vi "HEWH RLT PRAT.vi"() -> ()   [LabVIEW 2023] (continued)
"Condition#"=enum."C1", "Draw Flags"=enum."N/A", "Data Processing Delay (FHD 15sec, UEF 5 Sec)"=0.0, "Test Complete"=FALSE, "User Setpoint"=0.0, "Tank Setpoint"=0.0}, {"Sequence #"=6.0, "Cycles"=15, "Mode Setting"="", "Flow Rate (GPM)"=0.0, "Temperature (F)"=0.0, "Reset Timer"=FALSE, "Use Temp Decline Method"=FALSE, "Terminate Condition"=enum."C1-Terminate Draw @ Gallon Mark", "Condition Value #1"=0.0, "UE"=FALSE, "LE"=FALSE, "Comp"=FALSE, "Fan"=FALSE, "Test End Time (Sec)"=0.0, "Purge Until Cutout"=FALSE, "Start Conditions"=enum."Heat Source Cutout", "Condition Value #2"=0.0, "Remove Power"=FALSE, "Time"=0.0, "Check Special Cond."=enum."SC2-Check Heat Source (On-C2/Off-C1)", "Condition#"=enum."C1", "Draw Flags"=enum."N/A", "Data Processing Delay (FHD 15sec, UEF 5 Sec)"=0.0, "Test Complete"=FALSE, "User Setpoint"=0.0, "Tank Setpoint"=0.0}, {"Sequence #"=7.0, "Cycles"=35, "Mode Setting"="", "Flow Rate (GPM)"=0.0, "Temperature (F)"=0.0, "Reset Timer"=FALSE, "Use Temp Decline Method"=FALSE, "Terminate Condition"=enum."C1-Terminate Draw @ Gallon Mark", "Condition Value #1"=0.0, "UE"=FALSE, "LE"=FALSE, "Comp"=FALSE, "Fan"=FALSE, "Test End Time (Sec)"=0.0, "Purge Until Cutout"=FALSE, "Start Conditions"=enum."Heat Source Cutout", "Condition Value #2"=0.0, "Remove Power"=FALSE, "Time"=0.0, "Check Special Cond."=enum."SC2-Check Heat Source (On-C2/Off-C1)", "Condition#"=enum."C1", "Draw Flags"=enum."N/A", "Data Processing Delay (FHD 15sec, UEF 5 Sec)"=0.0, "Test Complete"=FALSE, "User Setpoint"=0.0, "Tank Setpoint"=0.0}, {"Sequence #"=8.0, "Cycles"=15, "Mode Setting"="", "Flow Rate (GPM)"=0.0, "Temperature (F)"=0.0, "Reset Timer"=FALSE, "Use Temp Decline Method"=FALSE, "Terminate Condition"=enum."C1-Terminate Draw @ Gallon Mark", "Condition Value #1"=0.0, "UE"=FALSE, "LE"=FALSE, "Comp"=FALSE, "Fan"=FALSE, "Test End Time (Sec)"=0.0, "Purge Until Cutout"=FALSE, "Start Conditions"=enum."Heat Source Cutout", "Condition Value #2"=0.0, "Remove Power"=FALSE, "Time"=0.0, "Check Special Cond."=enum."SC2-Check Heat Source (On-C2/Off-C1)", "Condition#"=enum."C1", "Draw Flags"=enum."N/A", "Data Processing Delay (FHD 15sec, UEF 5 Sec)"=0.0, "Test Complete"=FALSE, "User Setpoint"=0.0, "Tank Setpoint"=0.0}], "Current Sequence Index"=0}, "HEWH Specific DAQ"={"HEWH Data"={"HEWH Standard"={"Voltage (Volts)"=-1.0, "Current (Amps)"=-1.0, "Power (Watts)"=-1.0, "WattHours (Wh)"=-1.0, "TC Tree (AVG)"=0.0, "Flow Rate (GPM)"=0.0, "Gallons (Gal)"=0.0, "RTD Out (Deg F)"=0.0, "RTD In (Deg F)"=0.0, "RTD Amb (Deg F)"=0.0, "TC Down"=0.0, "UE Event Lead"=0, "LE Event Lead"=0, "TC 8"=0.0, "TC 9"=0.0, "TC 10"=0.0, "TC Tree Array (1-6)"=[], "TC 7"=0.0, "PSI 1"=0.0, "PSI 2"=0.0, "PSI 3"=0.0, "PSI 4"=0.0}, "PRAT"={"Power (Watts) A"=4192.0, "Power (Watts) B"=4192.0, "Power (Watts) C"=4192.0, "Power (Watts) D"=4192.0, "TC1"=0.0, "TC2"=0.0, "TC3"=0.0, "TC4"=0.0, "WattHours (Wh) A"=4192.0, "WattHours (Wh) B"=4192.0, "WattHours (Wh) C"=4192.0, "WattHours (Wh) D"=4192.0, "Ambient"=0.0, "Extra Temp"=0.0}, "Additional Power Data"={"Vthd"=236.2, "Frequency (Hz)"=236.2, "Apparent Power (VA)"=236.2, "Power Factor"=236.2, "Current Crest Factor"=236.2, "Voltage Crest Factor"=236.2, "Integration Time (sec)"=236.2}}, "Flow Valve % Open"=0.0, "Power State"={"UE"=FALSE, "LE"=FALSE, "COMP"=FALSE, "FANS"=FALSE}, "Power Analyzer"=enum."APLUS", "Flow Valve uA Output"=0, "Gallons Start (Gal)"=0.0, "PI Output"=0.0}, "Test Output Data"={"PreDraw Data Table"=[], "Data Table"=[], "MW100 TC Headers"=[]}, "Calc and Calibration"={"Mean SD Var Max Min Array"=[], "Draw Statistics (DBL)"=[], "Calibration Coefficients DBL"=[], "Start Gallons"=0.0, "Starting Temp Decline"=1000.0, "K-Factor (Temperature)"=0.0, "All Draw Stats"=[], "RTD Terminate Value"=0.0, "K-Factor (Flow)"=0.0, "Intellifaucet Type"="", "Thermal Stabil Array"=[], "Gas Thermal Stabil Complete"=FALSE, "Therm Reset Cmpt 1"=FALSE, "Therm Reset Cmpt 2"=FALSE, "Last Flow Rate (Therm)"=0.0, "State"=enum."State 1", "Gas Thermal Time"=0.0, "Target Rate (Thermal)"=0.0, "Thermal - Final"=[], "State5 Gal Water"=0.0, "State 5 Gal Gas"=0.0, "Intellif Open < 1"=0.0, "Intellif Open < 1.7"=0.0, "Intellif Open < 2.2"=0.0, "Intellif Open > 2.2"=0.0, "End of Draw\nComparison"=[], "Temperature Decline Method"={"Previous Cycle Count"=0, "Previous Max Temp In"=0.0, "Previous Trigger In"=0, "Start Timer"=0.0, "first_iteration"=0.0}}, "Current Draw Time"=0.0, "LV Program"=enum."HEWH", "Station ID"=enum."A", "Current Cond"=enum."N/A", "Test Complete"=FALSE, "ANSI Rate"={"Array 1"=[], "Array 3"=[], "Array 2"=[], "Start ANSI"=FALSE, "ANSI Start Time"=0.0, "Restart ANSI"=FALSE, "15 Min ANSI Avg (BTU/hr)"=0.0, "20 Min ANSI Avg (BTU/hr)"=0.0, "25 Min ANSI Avg (BTU/hr)"=0.0, "Absolute Pressure"=0.0, "Gas Temperature"=0.0, "Volumetric Flow Rate"=0.0, "Mass Flow Rate"=0.0, "Array 4"=[], "Array 5"=[], "Gas Rate"=0.0, "15 Min Pres Avg (PSIA)"=0.0, "20 Min Pres Avg (PSIA)"=0.0, "25 Min Pres Avg (PSIA)"=0.0, "15 Min Temp Avg (°F) "=0.0, "20 Min Temp Avg (°F)"=0.0, "25 Min Temp Avg (°F)"=0.0, "15 Min Uncorrected Avg (CFH)"=0.0, "20 Min Uncorrected Avg (CFH)"=0.0, "25 Min Uncorrected Avg (CFH)"=0.0, "15 Min Corrected Avg (SCFH)"=0.0, "20 Min Corrected Avg (SCFH)"=0.0, "25 Min Corrected Avg (SCFH)"=0.0, "15 Min Complete"=FALSE, "20 Min Complete"=FALSE, "25 Min Complete"=FALSE, "Heating Value (BTU/ft³)"=0.0, "CO CO2 15 Min"=[], "CO CO2 20 Min"=[], "CO CO2 25 Min"=[], "CO CO2 Real Time"=[]}, "Module 4 Relay Status"={"INTELLIFAUCET TEMP(T)/FLOW(F) (CH 041)"=FALSE, "INTELLIFAUCET READY (CH 042)"=FALSE, "INTELLIFAUCET START (CH 043)"=FALSE, "INTELLIFAUCET STOP (CH 044)"=FALSE, "MAIN POWER RELAY (CH 047)"=FALSE, "NOT USED (CH 045)"=FALSE, "NOT USED (CH 046)"=FALSE, "PURGE VALVE RELAY (CH 048)"=FALSE, "OUTLET VALVE RELAY (CH 049)"=FALSE, "INLET VALVE RELAY (CH 050)"=FALSE, "Intellifaucet (% Open)"=0.0, "Proportioning Valve (%Open)"=0.0, "Intellifaucet Temp Setpoint (F)"=0.0}} {"Test Patten Setup"."PRAT/RLT Sequence"."Time" format="%<%H:%M:%S>t"; "Test Patten Setup"."Total Gallons Schedule" format="%.2f"}
  out "File  Version":string="Parametric Stand"
  out "Software Elapsed Time":T29 format="%<%H:%M:%S>t"
  out "Message":T8
  in  "Start/Pause test":bool
  in  "Tab Control":T30(tab)
  in  "GEA2_D?":bool
  in  "GEA2_C?":bool
  in  "GEA2_B?":bool
  in  "GEA2_A?":bool
  out "Message D":string
  out "Message B":string
  out "Message C":string
  in  "New File Per CycD":bool
  in  "Reset Timer (D)":bool
  in  "New File Per CycC":bool
  in  "Reset Timer (C)":bool
  in  "New File Per CycB":bool
  in  "Reset Timer (B)":bool
  in  "New File Per CycA":bool
  in  "Reset Timer (A)":bool
  in  "StationD Setpoint":i32=140 caption="Unit Setpoint"
  in  "Cutout Delay D (sec)":dbl=240.0
  in  "StationC Setpoint":i32=140 caption="Unit Setpoint"
  in  "Cutout Delay C (sec)":dbl=240.0
  in  "StationB Setpoint":i32=140 caption="Unit Setpoint"
  in  "Cutout Delay B (sec)":dbl=240.0
  in  "StationA Setpoint":i32=140 caption="Unit Setpoint"
  in  "Cutout Delay A (sec)":dbl=240.0
  in  "Trigger Draw D":bool
  out "Remaining Draws (D)":i32=1000
  in  "Station D Display":T31={"Appliance Details"={"FileVersionInfo"={"FileVersion"="", "ProductName"="", "InternalName"="", "CompanyName"="", "LegalCopyright"="", "FileDescription"=""}, "Dishwasher Info"={"Open Cup Weight (gm):"=0.0, "Auto Cup Weight (gm):"=0.0, "Detergent-Dish:"="", "Inlet Temperature-Dish:"="", "Cycle Mode-Dish:"="", "Unit Control-Dish:"="", "Manufacturer-Dish:"=""}, "Washer Info"={"Hot Water Temperature (Fahrenheit):"="", "Cold Water Temperature (Fahrenheit):"="", "Capacity (cu.ft):"=0.0, "Initial Cloth Weight:"=0.0, "Cloth Lot:"=0, "Model Family:"="", "Program Name:"="", "Cycle Selection:"="", "Wash Temperature:"="", "Rinse Temperature:"="", "Load Size:"=""}, "File Name Output Array"=[], "Calibration Output Array"=[], "Appliance Common"={"Engineer:"="", "Model Number:"="", "Serial Number:"="", "Comments:"="", "Station ID:"="", "Technician:"="", "TR Number:"="", "Lab ID:"="", "Voltage:"="", "Water Pressure (PSI):"="", "Test Date:"="", "Computer Name:"="", "IP Address:"="", "Ambient RH:"="", "Frequency:"="", "Build:"="", "Filename:"="", "Test Type:"="", "Load Run #:"=0, "Ambient Temperature (F):"="", "File Path:"=path "", "Cycles Per Year"=60}, "Water Heater"={"Heating Mode:"=""}, "Dryer"={"Heat Setting:"="", "Washer Water Temperature (60 ± 5°F):"=60, "Water Hardness (PPM):"=17, "Dryness Setting:"="", "Dryer Type:"="", "Exhaust:"="", "Drying Cycle:"="", "Load Type:"="", "Nominal Load Weight"="", "Dryer Initial IMC Data"={"Measured IMC (lbs)"=7.0, "Actual Initial RMC (%)"=7.0, "RMC (Desired %)"=100.0, "Bone Dry Wt(lbs)"=7.0, "Tolerance(%)"=5.0, "Actual Final RMC (%)"=0.0, "CEF (lbf/kWh)"=0.0, "Minimum Weight (lbf)"=0.0, "Average Weight (lbf)"=0.0, "Maximum Weight (lbf)"=0.0, "Measured IMC In Range?"=FALSE, "Moisture Reduction Factor"=55.5, "Field Use Factor"=1.04, "Empty Dryer Cold Weigth"=0.0, "Energy Standard"=enum."D2-Automatic Dryer", "Weight Cloth (lbs)"=0.0, "Relative Moisture Content (%)"=0.0, "Relative Moisture Content - Avg (%)"=0.0}}}, "Display Data (RLT)"={"Status Color"=0, "Serial Number Display"="", "Cycle Count Display"=0, "Station Label Display"="", "Current Run Start Time Display"=0.0, "Board ID Display"="", "RPM Display"=0, "Current Display"=0.0, "Current Path Display"=path "", "Saving Display"=FALSE, "Unit Type Display"=enum."", "Total Time On Display"=0.0, "UI Button"=FALSE}} {"Display Data (RLT)"."Current Display" format="%.2f"; "Display Data (RLT)"."Cycle Count Display" format="%04d"; "Appliance Details"."Dryer"."Dryer Initial IMC Data"."Maximum Weight (lbf)" format="%03_6g"; "Appliance Details"."Dryer"."Dryer Initial IMC Data"."Average Weight (lbf)" format="%03_6g"; "Appliance Details"."Dryer"."Dryer Initial IMC Data"."Minimum Weight (lbf)" format="%03_6g"; "Appliance Details"."Dryer"."Dryer Initial IMC Data"."CEF (lbf/kWh)" format="%03_6g"; "Appliance Details"."Dryer"."Dryer Initial IMC Data"."Actual Final RMC (%)" format="%03_6g"; "Appliance Details"."Dryer"."Dryer Initial IMC Data"."Tolerance(%)" format="%0#_6g"; "Appliance Details"."Dryer"."Dryer Initial IMC Data"."Bone Dry Wt(lbs)" format="%03_6g"; "Appliance Details"."Dryer"."Dryer Initial IMC Data"."RMC (Desired %)" format="%0#_6g"; "Appliance Details"."Dryer"."Dryer Initial IMC Data"."Actual Initial RMC (%)" format="%03_6g"; "Appliance Details"."Dryer"."Dryer Initial IMC Data"."Measured IMC (lbs)" format="%0#_6g"}
  in  "DAQ for D":bool
  out "POWERD":T23
  out "Degree Setting( Station D)":dbl=58.0 caption="Degree Setting( F)"
  out "Draw Amount (Station D)":dbl=15.0 caption="Draw Amount (Gal)"
  out "GPM Target (Station D)":dbl=3.0 caption="GPM Target"
  out "Station D":string[][](array[string])
  in  "Disable Station 4":T34
  in  "Trigger Draw B":bool
  out "Remaining Draws (B)":i32=1000
  in  "Station B Display":T31={"Appliance Details"={"FileVersionInfo"={"FileVersion"="", "ProductName"="", "InternalName"="", "CompanyName"="", "LegalCopyright"="", "FileDescription"=""}, "Dishwasher Info"={"Open Cup Weight (gm):"=0.0, "Auto Cup Weight (gm):"=0.0, "Detergent-Dish:"="", "Inlet Temperature-Dish:"="", "Cycle Mode-Dish:"="", "Unit Control-Dish:"="", "Manufacturer-Dish:"=""}, "Washer Info"={"Hot Water Temperature (Fahrenheit):"="", "Cold Water Temperature (Fahrenheit):"="", "Capacity (cu.ft):"=0.0, "Initial Cloth Weight:"=0.0, "Cloth Lot:"=0, "Model Family:"="", "Program Name:"="", "Cycle Selection:"="", "Wash Temperature:"="", "Rinse Temperature:"="", "Load Size:"=""}, "File Name Output Array"=[], "Calibration Output Array"=[], "Appliance Common"={"Engineer:"="", "Model Number:"="", "Serial Number:"="", "Comments:"="", "Station ID:"="", "Technician:"="", "TR Number:"="", "Lab ID:"="", "Voltage:"="", "Water Pressure (PSI):"="", "Test Date:"="", "Computer Name:"="", "IP Address:"="", "Ambient RH:"="", "Frequency:"="", "Build:"="", "Filename:"="", "Test Type:"="", "Load Run #:"=0, "Ambient Temperature (F):"="", "File Path:"=path "", "Cycles Per Year"=60}, "Water Heater"={"Heating Mode:"=""}, "Dryer"={"Heat Setting:"="", "Washer Water Temperature (60 ± 5°F):"=60, "Water Hardness (PPM):"=17, "Dryness Setting:"="", "Dryer Type:"="", "Exhaust:"="", "Drying Cycle:"="", "Load Type:"="", "Nominal Load Weight"="", "Dryer Initial IMC Data"={"Measured IMC (lbs)"=7.0, "Actual Initial RMC (%)"=7.0, "RMC (Desired %)"=100.0, "Bone Dry Wt(lbs)"=7.0, "Tolerance(%)"=5.0, "Actual Final RMC (%)"=0.0, "CEF (lbf/kWh)"=0.0, "Minimum Weight (lbf)"=0.0, "Average Weight (lbf)"=0.0, "Maximum Weight (lbf)"=0.0, "Measured IMC In Range?"=FALSE, "Moisture Reduction Factor"=55.5, "Field Use Factor"=1.04, "Empty Dryer Cold Weigth"=0.0, "Energy Standard"=enum."D2-Automatic Dryer", "Weight Cloth (lbs)"=0.0, "Relative Moisture Content (%)"=0.0, "Relative Moisture Content - Avg (%)"=0.0}}}, "Display Data (RLT)"={"Status Color"=0, "Serial Number Display"="", "Cycle Count Display"=0, "Station Label Display"="", "Current Run Start Time Display"=0.0, "Board ID Display"="", "RPM Display"=0, "Current Display"=0.0, "Current Path Display"=path "", "Saving Display"=FALSE, "Unit Type Display"=enum."", "Total Time On Display"=0.0, "UI Button"=FALSE}} {"Display Data (RLT)"."Current Display" format="%.2f"; "Display Data (RLT)"."Cycle Count Display" format="%04d"; "Appliance Details"."Dryer"."Dryer Initial IMC Data"."Maximum Weight (lbf)" format="%03_6g"; "Appliance Details"."Dryer"."Dryer Initial IMC Data"."Average Weight (lbf)" format="%03_6g"; "Appliance Details"."Dryer"."Dryer Initial IMC Data"."Minimum Weight (lbf)" format="%03_6g"; "Appliance Details"."Dryer"."Dryer Initial IMC Data"."CEF (lbf/kWh)" format="%03_6g"; "Appliance Details"."Dryer"."Dryer Initial IMC Data"."Actual Final RMC (%)" format="%03_6g"; "Appliance Details"."Dryer"."Dryer Initial IMC Data"."Tolerance(%)" format="%0#_6g"; "Appliance Details"."Dryer"."Dryer Initial IMC Data"."Bone Dry Wt(lbs)" format="%03_6g"; "Appliance Details"."Dryer"."Dryer Initial IMC Data"."RMC (Desired %)" format="%0#_6g"; "Appliance Details"."Dryer"."Dryer Initial IMC Data"."Actual Initial RMC (%)" format="%03_6g"; "Appliance Details"."Dryer"."Dryer Initial IMC Data"."Measured IMC (lbs)" format="%0#_6g"}
  in  "DAQ for B":bool
  out "POWERB":T23
  out "Degree Setting( Station B)":dbl=58.0 caption="Degree Setting( F)"
  out "GPM Target (Station B)":dbl=3.0 caption="GPM Target"
  out "Draw Amount (Station B)":dbl=15.0 caption="Draw Amount (Gal)"
  out "Station B":string[][](array[string])
  in  "Disable Station 2":T34
  in  "Trigger Draw A":bool
  out "Remaining Draws (A)":i32=1000
  out "Message A":string
  in  "DAQ for A":bool
  in  "Disable Station 1":T34
  out "Draw Amount (Station A)":dbl=15.0 caption="Draw Amount (Gal)"
  out "GPM Target (Station A)":dbl=3.0 caption="GPM Target"
  out "Degree Setting( Station A)":dbl=58.0 caption="Degree Setting( F)"
  in  "Station A Display":T31={"Appliance Details"={"FileVersionInfo"={"FileVersion"="", "ProductName"="", "InternalName"="", "CompanyName"="", "LegalCopyright"="", "FileDescription"=""}, "Dishwasher Info"={"Open Cup Weight (gm):"=0.0, "Auto Cup Weight (gm):"=0.0, "Detergent-Dish:"="", "Inlet Temperature-Dish:"="", "Cycle Mode-Dish:"="", "Unit Control-Dish:"="", "Manufacturer-Dish:"=""}, "Washer Info"={"Hot Water Temperature (Fahrenheit):"="", "Cold Water Temperature (Fahrenheit):"="", "Capacity (cu.ft):"=0.0, "Initial Cloth Weight:"=0.0, "Cloth Lot:"=0, "Model Family:"="", "Program Name:"="", "Cycle Selection:"="", "Wash Temperature:"="", "Rinse Temperature:"="", "Load Size:"=""}, "File Name Output Array"=[], "Calibration Output Array"=[], "Appliance Common"={"Engineer:"="", "Model Number:"="", "Serial Number:"="", "Comments:"="", "Station ID:"="", "Technician:"="", "TR Number:"="", "Lab ID:"="", "Voltage:"="", "Water Pressure (PSI):"="", "Test Date:"="", "Computer Name:"="", "IP Address:"="", "Ambient RH:"="", "Frequency:"="", "Build:"="", "Filename:"="", "Test Type:"="", "Load Run #:"=0, "Ambient Temperature (F):"="", "File Path:"=path "", "Cycles Per Year"=60}, "Water Heater"={"Heating Mode:"=""}, "Dryer"={"Heat Setting:"="", "Washer Water Temperature (60 ± 5°F):"=60, "Water Hardness (PPM):"=17, "Dryness Setting:"="", "Dryer Type:"="", "Exhaust:"="", "Drying Cycle:"="", "Load Type:"="", "Nominal Load Weight"="", "Dryer Initial IMC Data"={"Measured IMC (lbs)"=7.0, "Actual Initial RMC (%)"=7.0, "RMC (Desired %)"=100.0, "Bone Dry Wt(lbs)"=7.0, "Tolerance(%)"=5.0, "Actual Final RMC (%)"=0.0, "CEF (lbf/kWh)"=0.0, "Minimum Weight (lbf)"=0.0, "Average Weight (lbf)"=0.0, "Maximum Weight (lbf)"=0.0, "Measured IMC In Range?"=FALSE, "Moisture Reduction Factor"=55.5, "Field Use Factor"=1.04, "Empty Dryer Cold Weigth"=0.0, "Energy Standard"=enum."D2-Automatic Dryer", "Weight Cloth (lbs)"=0.0, "Relative Moisture Content (%)"=0.0, "Relative Moisture Content - Avg (%)"=0.0}}}, "Display Data (RLT)"={"Status Color"=0, "Serial Number Display"="", "Cycle Count Display"=0, "Station Label Display"="", "Current Run Start Time Display"=0.0, "Board ID Display"="", "RPM Display"=0, "Current Display"=0.0, "Current Path Display"=path "", "Saving Display"=FALSE, "Unit Type Display"=enum."", "Total Time On Display"=0.0, "UI Button"=FALSE}} {"Display Data (RLT)"."Current Display" format="%.2f"; "Display Data (RLT)"."Cycle Count Display" format="%04d"; "Appliance Details"."Dryer"."Dryer Initial IMC Data"."Maximum Weight (lbf)" format="%03_6g"; "Appliance Details"."Dryer"."Dryer Initial IMC Data"."Average Weight (lbf)" format="%03_6g"; "Appliance Details"."Dryer"."Dryer Initial IMC Data"."Minimum Weight (lbf)" format="%03_6g"; "Appliance Details"."Dryer"."Dryer Initial IMC Data"."CEF (lbf/kWh)" format="%03_6g"; "Appliance Details"."Dryer"."Dryer Initial IMC Data"."Actual Final RMC (%)" format="%03_6g"; "Appliance Details"."Dryer"."Dryer Initial IMC Data"."Tolerance(%)" format="%0#_6g"; "Appliance Details"."Dryer"."Dryer Initial IMC Data"."Bone Dry Wt(lbs)" format="%03_6g"; "Appliance Details"."Dryer"."Dryer Initial IMC Data"."RMC (Desired %)" format="%0#_6g"; "Appliance Details"."Dryer"."Dryer Initial IMC Data"."Actual Initial RMC (%)" format="%03_6g"; "Appliance Details"."Dryer"."Dryer Initial IMC Data"."Measured IMC (lbs)" format="%0#_6g"}
  out "POWERA":T23
  out "Station A":string[][](array[string])
  in  "Trigger Draw C":bool
  out "Remaining Draws (C)":i32=1000
  in  "Station C Display":T31={"Appliance Details"={"FileVersionInfo"={"FileVersion"="", "ProductName"="", "InternalName"="", "CompanyName"="", "LegalCopyright"="", "FileDescription"=""}, "Dishwasher Info"={"Open Cup Weight (gm):"=0.0, "Auto Cup Weight (gm):"=0.0, "Detergent-Dish:"="", "Inlet Temperature-Dish:"="", "Cycle Mode-Dish:"="", "Unit Control-Dish:"="", "Manufacturer-Dish:"=""}, "Washer Info"={"Hot Water Temperature (Fahrenheit):"="", "Cold Water Temperature (Fahrenheit):"="", "Capacity (cu.ft):"=0.0, "Initial Cloth Weight:"=0.0, "Cloth Lot:"=0, "Model Family:"="", "Program Name:"="", "Cycle Selection:"="", "Wash Temperature:"="", "Rinse Temperature:"="", "Load Size:"=""}, "File Name Output Array"=[], "Calibration Output Array"=[], "Appliance Common"={"Engineer:"="", "Model Number:"="", "Serial Number:"="", "Comments:"="", "Station ID:"="", "Technician:"="", "TR Number:"="", "Lab ID:"="", "Voltage:"="", "Water Pressure (PSI):"="", "Test Date:"="", "Computer Name:"="", "IP Address:"="", "Ambient RH:"="", "Frequency:"="", "Build:"="", "Filename:"="", "Test Type:"="", "Load Run #:"=0, "Ambient Temperature (F):"="", "File Path:"=path "", "Cycles Per Year"=60}, "Water Heater"={"Heating Mode:"=""}, "Dryer"={"Heat Setting:"="", "Washer Water Temperature (60 ± 5°F):"=60, "Water Hardness (PPM):"=17, "Dryness Setting:"="", "Dryer Type:"="", "Exhaust:"="", "Drying Cycle:"="", "Load Type:"="", "Nominal Load Weight"="", "Dryer Initial IMC Data"={"Measured IMC (lbs)"=7.0, "Actual Initial RMC (%)"=7.0, "RMC (Desired %)"=100.0, "Bone Dry Wt(lbs)"=7.0, "Tolerance(%)"=5.0, "Actual Final RMC (%)"=0.0, "CEF (lbf/kWh)"=0.0, "Minimum Weight (lbf)"=0.0, "Average Weight (lbf)"=0.0, "Maximum Weight (lbf)"=0.0, "Measured IMC In Range?"=FALSE, "Moisture Reduction Factor"=55.5, "Field Use Factor"=1.04, "Empty Dryer Cold Weigth"=0.0, "Energy Standard"=enum."D2-Automatic Dryer", "Weight Cloth (lbs)"=0.0, "Relative Moisture Content (%)"=0.0, "Relative Moisture Content - Avg (%)"=0.0}}}, "Display Data (RLT)"={"Status Color"=0, "Serial Number Display"="", "Cycle Count Display"=0, "Station Label Display"="", "Current Run Start Time Display"=0.0, "Board ID Display"="", "RPM Display"=0, "Current Display"=0.0, "Current Path Display"=path "", "Saving Display"=FALSE, "Unit Type Display"=enum."", "Total Time On Display"=0.0, "UI Button"=FALSE}} {"Display Data (RLT)"."Current Display" format="%.2f"; "Display Data (RLT)"."Cycle Count Display" format="%04d"; "Appliance Details"."Dryer"."Dryer Initial IMC Data"."Maximum Weight (lbf)" format="%03_6g"; "Appliance Details"."Dryer"."Dryer Initial IMC Data"."Average Weight (lbf)" format="%03_6g"; "Appliance Details"."Dryer"."Dryer Initial IMC Data"."Minimum Weight (lbf)" format="%03_6g"; "Appliance Details"."Dryer"."Dryer Initial IMC Data"."CEF (lbf/kWh)" format="%03_6g"; "Appliance Details"."Dryer"."Dryer Initial IMC Data"."Actual Final RMC (%)" format="%03_6g"; "Appliance Details"."Dryer"."Dryer Initial IMC Data"."Tolerance(%)" format="%0#_6g"; "Appliance Details"."Dryer"."Dryer Initial IMC Data"."Bone Dry Wt(lbs)" format="%03_6g"; "Appliance Details"."Dryer"."Dryer Initial IMC Data"."RMC (Desired %)" format="%0#_6g"; "Appliance Details"."Dryer"."Dryer Initial IMC Data"."Actual Initial RMC (%)" format="%03_6g"; "Appliance Details"."Dryer"."Dryer Initial IMC Data"."Measured IMC (lbs)" format="%0#_6g"}
  in  "DAQ for C":bool
  out "POWERC":T23
  out "Degree Setting( Station C)":dbl=58.0 caption="Degree Setting( F)"
  out "GPM Target (Station C)":dbl=3.0 caption="GPM Target"
  out "Draw Amount (Station C)":dbl=15.0 caption="Draw Amount (Gal)"
  out "Station C":string[][](array[string])
  in  "Disable Station 3":T34
  in  "Proportioning\nValve":dbl(slide) min=0.0 max=100.0 scale=0.0..100.0
  in  "Valve % Open":dbl(slide) min=0.0 max=100.0 scale=0.0..100.0
  in  "Temp (°F)":dbl(slide)=58.0 min=32.0 max=203.0 scale=40.0..140.0
  in  "IF Start":bool
  in  "IF Stop":bool
  in  "Reset Power Analyzer":bool
  in  "Tab Control 4":T35(tab)
  in  "Show Stand Override Flow Data A":bool
  in  "Y-Axis2 - Station A":string(combo)
  in  "Y-Axis1 - Station A":string(combo)
  in  "X-Axis - Station A":string(combo)
  in  "Clear Graph Data":bool
  in  "Pause Graph":bool
  out "Station A SO Display":string[][](array[string])
  out "Tank Display - Station A":T36 {"TC6" format="%.2g"; "TIN" format="%.2g"; "TOUT" format="%.2g"; "TC5" format="%.2g"; "TC4" format="%.2g"; "TC3" format="%.2g"; "TC2" format="%.2g"; "TC1" format="%.2g"}
  out "XY Graph - Station A":T37(graph)
  out "POWERA Display":T23
  out "Test Procedure":string
  out "Timer 1":string
  in  "X-Axis - Station B":string(combo)
  in  "Y-Axis1 - Station B":string(combo)
  in  "Y-Axis2 - Station B":string(combo)
  out "XY Graph - Station B":T37(graph)
  out "Tank Display - Station B":T36 {"TC6" format="%.2g"; "TIN" format="%.2g"; "TOUT" format="%.2g"; "TC5" format="%.2g"; "TC4" format="%.2g"; "TC3" format="%.2g"; "TC2" format="%.2g"; "TC1" format="%.2g"}
  in  "Clear Graph Data B":bool caption="Clear Graph Data"
  in  "Pause Graph B":bool caption="Pause Graph"
  out "Station B SO Display":string[][](array[string])
  in  "Show Stand Override Flow Data B":bool
  out "POWERB Display":T23
  out "Test Procedure 2":string
  out "Timer 2":string
  in  "X-Axis - Station C":string(combo)
  in  "Y-Axis1 - Station C":string(combo)
  in  "Y-Axis2 - Station C":string(combo)
  out "Tank Display - Station C":T36 {"TC6" format="%.2g"; "TIN" format="%.2g"; "TOUT" format="%.2g"; "TC5" format="%.2g"; "TC4" format="%.2g"; "TC3" format="%.2g"; "TC2" format="%.2g"; "TC1" format="%.2g"}
  in  "Clear Graph Data C":bool caption="Clear Graph Data"
  in  "Pause Graph C":bool caption="Pause Graph"
  out "XY Graph - Station C":T37(graph)
  out "Station C SO Display":string[][](array[string])
  in  "Show Stand Override Flow Data C":bool
  out "POWERC Display":T23
  out "Test Procedure 3":string
  out "Timer 3":string
  in  "X-Axis - Station D":string(combo)
  in  "Y-Axis1 - Station D":string(combo)
  in  "Y-Axis2 - Station D":string(combo)
  out "XY Graph - Station D":T37(graph)
  out "Tank Display - Station D":T36 {"TC6" format="%.2g"; "TIN" format="%.2g"; "TOUT" format="%.2g"; "TC5" format="%.2g"; "TC4" format="%.2g"; "TC3" format="%.2g"; "TC2" format="%.2g"; "TC1" format="%.2g"}
  in  "Clear Graph Data D":bool caption="Clear Graph Data"
  in  "Pause Graph D":bool caption="Pause Graph"
  out "Station D SO Display":string[][](array[string])
  in  "Show Stand Override Flow Data D":bool
  out "POWERD Display":T23
  out "Test Procedure 4":string
  out "Timer 4":string
  in  "Cancel Draw":bool
  in  "Main Power":bool
  in  "Pressurize Tank?":bool=TRUE
  in  "Skip Purge":bool
  in  "Skip Draw":bool
  in  "Tab Control 5":T38(tab)
  in  "Set Valves-D":bool
  in  "Station D Valve Setting":T39
  in  "Set Valves-C":bool
  in  "Station C Valve Setting":T39
  in  "Set Valves-B":bool
  in  "Station B Valve Setting":T39
  in  "Set Valves-A":bool
  in  "Proportioning Valve Upper Limit":dbl=100.0
  in  "Proportioning Valve Step Time (Sec)":i16=5 min=1
  in  "AUTO STEP":bool
  in  "Auto Step Increment":dbl=0.067
  in  "Station A Valve Setting":T39
  in  "Outlet Valve D":T40="ON"
  in  "Drain Valve D":T41="OFF"
  in  "Inlet Valve D":T40="ON"
  in  "Outlet Valve C":T40="ON"
  in  "Drain Valve C":T41="OFF"
  in  "Inlet Valve C":T40="ON"
  in  "Outlet Valve B":T40="ON"
  in  "Drain Valve B":T41="OFF"
  in  "Inlet Valve B":T40="ON"
  in  "Outlet Valve A":T40="ON"
  in  "Drain Valve A":T41="OFF"
  in  "Inlet Valve A":T40="ON"
  out "Message A Detail":string
  out "Message B Detail":string
  out "Message C Detail":string
  out "Message D Detail":string
  in  "Update Capacity":bool
  in  "Reset Control Counter":bool
  in  "Update User Setpoint":bool
  in  "User Setpoint":i32=125 min=40 max=190 step=1
  in  "Heating Mode.":T16
  in  "Update Mode":bool
  in  "TankSP Offset":i16
  in  "Update TankSP Offset":bool
  in  "Update Personality":bool
  in  "Personality":T42
  in  "Capacity Setting":string(combo)
  in  "Enable EMV ERD List":bool
  in  "Enable Heat Pump ERD List":bool
  in  "Enable Inverter ERD List":bool
  out "Raw Timer Output":T29 format="%<%H:%M:%S>t"
  in  "Test Type - Rate":string(combo)="Rate"
  out "ANSI Display 1":string
  in  "Start ANSI UI":bool caption="Start ANSI"
  out "Rate Outputs":string[][](array[string])
  in  "Reset Totalizer":bool
  in  "Tare Meter":bool
  in  "Pilot Flow Rate (SCFH)":dbl=1.4
  in  "Gas Type":T43="189"
  in  "HHV-NG-Manual":sgl=1069.0
  in  "HHV-LP-Manual":sgl=2548.0
  in  "Manual Heating Value":bool
  in  "Ultramat  COM Port":refnum<visa-resource-name>
  in  "Update Vesta Temp":bool
  in  "Vesta COM Port":refnum<visa-resource-name>
  in  "Temperature Parameters":T44={"Water Heater Temp (°F)"=120, "Differential  (°F)"=10.0} {"Water Heater Temp (°F)" min=32 max=203}
  out "Connection Status Vesta":bool caption="Connection Status"
  in  "Burner Status":T45
  in  "Enviracom COM Port":refnum<visa-resource-name>
  in  "Update Enviracom Status":bool
  out "Connection Status Envira":bool caption="Connection Status"
  in  "Reset Flow Meter":bool
  in  "Reset Inventory":bool
  in  "Temperature Decline Amount (°F)":dbl=0.01
  in  "Purge Time (Seconds)":dbl=480.0
  in  "Pressurization Time (sec)":i32=5
  in  "NOx Purge Time":dbl=0.01
  in  "Tab Control 8":enum32{"Main", "Debug"}(tab)
  in  "Chamber Status":T46
  in  "Set Status":bool
  in  "Set Temperature":bool
  in  "Set Humidity":bool
  in  "Set Frequency":bool
  in  "Setpoint Temperature (F)":dbl=67.5 min=32.0 max=135.0
  in  "Setpoint Humidity (%)":dbl=50.0 min=0.0 max=100.0
  in  "Setpoint Frequency (Hz)":dbl=10.0 min=5.0 max=60.0
  in  "Temperature Limits":T47={"Target Temperature Upper limit"=68.75, "Target Temperature Lower limit"=67.75, "Target Humidity Lower limit"=48.5, "Target Humidity Upper limit"=50.5, "Chamber Temperature Upper limit"=73.0, "Chamber Temperature Lower limit"=63.0, "Chamber Humidity Lower limit"=40.0, "Chamber Humidity Upper limit"=55.0, "Chamber Adjustment Increment (F)"=0.25, "Chamber Adjustment Interval (Minutes)"=10.0, "Chamber Adjustment Increment (%)"=0.25, "Chamber Adjustment Interval Fast (Minutes)"=10.0}
  in  "Update Temperature Limits":bool
  in  "Enable Auto Control":bool
  in  "Sample Rate (mS)":u32=3000
  out "Viasala.Probe Number":u16
  out "Main Array":string[](array[string])
  in  "Enable Arrays":bool
  in  "Connect Tenney Counter":dbl
  in  "Connect Viasala Counter":dbl
  in  "Elapsed Time (Min)":dbl
  in  "Tenney Chamber Loop Counter":i32
  in  "Viasala Loop Counter":i32
  in  "Data Array":dbl[][](array[numeric])
  out "Tenney Array":string[](array[string])
  out "Viasala Array":string[](array[string])
  out "Current Draw Parameters":T48={"Draws Left"=0, "Draws Left Array"=[], "Remaining Draws (A)"=1000, "Remaining Draws (B)"=1000, "Remaining Draws (C)"=1000, "Remaining Draws (D)"=1000, "Index of Element (A-D)"=[], "Station A"={"Sequence #"=0.0, "Cycles"=0, "Mode Setting"="", "Flow Rate (GPM)"=0.0, "Temperature (F)"=0.0, "Reset Timer"=FALSE, "Use Temp Decline Method"=FALSE, "Terminate Condition"=enum."C1-Terminate Draw @ Gallon Mark", "Condition Value #1"=0.0, "UE"=FALSE, "LE"=FALSE, "Comp"=FALSE, "Fan"=FALSE, "Test End Time (Sec)"=0.0, "Purge Until Cutout"=FALSE, "Start Conditions"=enum."Heat Source Cutout", "Condition Value #2"=0.0, "Remove Power"=FALSE, "Time"=0.0, "Check Special Cond."=enum."SC2-Check Heat Source (On-C2/Off-C1)", "Condition#"=enum."C1", "Draw Flags"=enum."N/A", "Data Processing Delay (FHD 15sec, UEF 5 Sec)"=0.0, "Test Complete"=FALSE, "User Setpoint"=0.0, "Tank Setpoint"=0.0}, "Station B"={"Sequence #"=0.0, "Cycles"=0, "Mode Setting"="", "Flow Rate (GPM)"=0.0, "Temperature (F)"=0.0, "Reset Timer"=FALSE, "Use Temp Decline Method"=FALSE, "Terminate Condition"=enum."C1-Terminate Draw @ Gallon Mark", "Condition Value #1"=0.0, "UE"=FALSE, "LE"=FALSE, "Comp"=FALSE, "Fan"=FALSE, "Test End Time (Sec)"=0.0, "Purge Until Cutout"=FALSE, "Start Conditions"=enum."Heat Source Cutout", "Condition Value #2"=0.0, "Remove Power"=FALSE, "Time"=0.0, "Check Special Cond."=enum."SC2-Check Heat Source (On-C2/Off-C1)", "Condition#"=enum."C1", "Draw Flags"=enum."N/A", "Data Processing Delay (FHD 15sec, UEF 5 Sec)"=0.0, "Test Complete"=FALSE, "User Setpoint"=0.0, "Tank Setpoint"=0.0}, "Station C"={"Sequence #"=0.0, "Cycles"=0, "Mode Setting"="", "Flow Rate (GPM)"=0.0, "Temperature (F)"=0.0, "Reset Timer"=FALSE, "Use Temp Decline Method"=FALSE, "Terminate Condition"=enum."C1-Terminate Draw @ Gallon Mark", "Condition Value #1"=0.0, "UE"=FALSE, "LE"=FALSE, "Comp"=FALSE, "Fan"=FALSE, "Test End Time (Sec)"=0.0, "Purge Until Cutout"=FALSE, "Start Conditions"=enum."Heat Source Cutout", "Condition Value #2"=0.0, "Remove Power"=FALSE, "Time"=0.0, "Check Special Cond."=enum."SC2-Check Heat Source (On-C2/Off-C1)", "Condition#"=enum."C1", "Draw Flags"=enum."N/A", "Data Processing Delay (FHD 15sec, UEF 5 Sec)"=0.0, "Test Complete"=FALSE, "User Setpoint"=0.0, "Tank Setpoint"=0.0}, "Station D"={"Sequence #"=0.0, "Cycles"=0, "Mode Setting"="", "Flow Rate (GPM)"=0.0, "Temperature (F)"=0.0, "Reset Timer"=FALSE, "Use Temp Decline Method"=FALSE, "Terminate Condition"=enum."C1-Terminate Draw @ Gallon Mark", "Condition Value #1"=0.0, "UE"=FALSE, "LE"=FALSE, "Comp"=FALSE, "Fan"=FALSE, "Test End Time (Sec)"=0.0, "Purge Until Cutout"=FALSE, "Start Conditions"=enum."Heat Source Cutout", "Condition Value #2"=0.0, "Remove Power"=FALSE, "Time"=0.0, "Check Special Cond."=enum."SC2-Check Heat Source (On-C2/Off-C1)", "Condition#"=enum."C1", "Draw Flags"=enum."N/A", "Data Processing Delay (FHD 15sec, UEF 5 Sec)"=0.0, "Test Complete"=FALSE, "User Setpoint"=0.0, "Tank Setpoint"=0.0}} {"Station D"."Time" format="%<%H:%M:%S>t"; "Station C"."Time" format="%<%H:%M:%S>t"; "Station B"."Time" format="%<%H:%M:%S>t"; "Station A"."Time" format="%<%H:%M:%S>t"}
  in  "GEA3 Pink Bean Board Index (Station D)":T49=enum."Board ID - 3"
  in  "GEA3 Pink Bean Board Index (Station C)":T49=enum."Board ID - 2"
  in  "GEA3 Pink Bean Board Index (Station B)":T49=enum."Board ID - 1"
  in  "GEA3 Pink Bean Board Index (Station A)":T49
  in  "Station ID":T50
  in  "Range Configuration (True)":bool[](array[boolean])=[FALSE, FALSE, FALSE, FALSE, FALSE, TRUE, TRUE, TRUE, TRUE, TRUE, TRUE, TRUE, FALSE]
  in  "Tab Control 6":T35(tab)
  in  "File Locations A":T3
  in  "File Locations B":T3
  in  "File Locations C":T3
  in  "File Locations D":T3
  in  "Enable Auto Range (F: Disable)":bool=TRUE
  in  "Manual Range (20 <10> A)":dbl(ring)=10.0 items=["5m <2.5m>"=0.0025, "10m <5m>"=0.005, "20m <10m>"=0.01, "50m <25m>"=0.025, "100m <50m>"=0.05, "200m <100m>"=0.1, "500m <250m>"=0.25, "1 <500m>"=0.5, "2 <1>"=1.0, "5 <2.5>"=2.5, "10 <5>"=5.0, "20 <10>"=10.0, "40 <20>"=20.0]
  in  "MW100 COM Port":refnum<visa-resource-name>="MW100"
  in  "Agilent COM Port":refnum<visa-resource-name>="34972A"
  in  "Heise Barometer COM Port":refnum<visa-resource-name>="HEISE"
  in  "WT300 COM Port":refnum<visa-resource-name>="WT300"
  in  "Laurel IP Address":string="10.2.0.23"
  in  "Alicat COM Port":refnum<visa-resource-name>="Alicat"
  in  "Ritter COM Port":refnum<visa-resource-name>="Ritter"
  in  "Emerson IP Address":string="10.2.0.173"
  in  "NG Inficon IP Address":string="192.168.1.32"
  in  "LP Inficon IP Address":string="192.168.1.33"
  in  "Viasala IP Address":string
  in  "Tenney IP Address":string
  out "Shutdown":string="Stop Flow\nMacro: Exit"
  in  "Development Tab":T51(tab)
  out "Disable Purge Pressurization D":bool
  out "Disable Purge Pressurization C":bool
  out "Disable Purge Pressurization B":bool
  out "Final Headers D":bool
  out "Final Headers C":bool
  out "Final Headers B":bool
  out "Final Headers A":bool
  out "Use Last Start Condition D?":bool
  out "Use Last Start Condition C?":bool
  out "Use Last Start Condition B?":bool
  out "Finish":bool=TRUE
  in  "User Controls":T52={"Main Power Control"=FALSE, "Flow Totalizer Control"=FALSE, "Intellifaucet \nTemperature"=58.0, "Percent Flow"=0.0, "Safe Mode"=FALSE, "GEA2?"=TRUE, "Use Agilent?"=FALSE, "Valve Set A"=enum."Heating", "Valve Set B"=enum."Heating", "Valve Set C"=enum."Heating", "Valve Set D"=enum."Heating", "Valve Ctrl"={"Outlet Valve D"="OFF", "Drain Valve D"="OFF", "Inlet Valve D"="OFF", "Outlet Valve C"="OFF", "Drain Valve C"="OFF", "Inlet Valve C"="OFF", "Outlet Valve B"="OFF", "Drain Valve B"="OFF", "Inlet Valve B"="OFF", "Outlet Valve A"="OFF", "Drain Valve A"="OFF", "Inlet Valve A"="OFF"}, "Proportional Valve"=0.0, "Reset Auto Step"=FALSE} {"Proportional Valve" scale=0.0..100.0; "Percent Flow" scale=0.0..100.0; "Intellifaucet \nTemperature" scale=40.0..120.0}
  out "Station ID to Reset":T26=enum."A"
  out "Draws Left":i32
  out "Error Out":errorcluster
  in  "Error In":errorcluster
  out "Draw Loop":i32
  out "Draw Complete":bool
  out "MW100":refnum<visa-resource-name>
  out "Start Draw Loop":bool
  out "Draw Station":string
  in  "File Locations In":T3
  in  "Tab Control 3":enum32{"A", "B", "C", "D"}(tab)
  out "DAQ Finished":bool=TRUE
  out "GEA3 Read Message Loop":i32
  out "K-Factor (Temperature)":dbl=100.0
  out "LV Program":T25
  out "A Timer":dbl
  out "B Timer":dbl
  out "C Timer":dbl
  out "D Timer":dbl
  out "Temp Decline Complete A":bool
  out "Temp Decline Complete B":bool
  out "Temp Decline Complete C":bool
  out "Temp Decline Complete D":bool
  out "Yokogawa WT210":refnum<visa-resource-name>
  out "Use Last Start Condition A?":bool
  out "Log Data Output (D)":bool
  out "Log Data Output (A)":bool
  out "Log Data Output (B)":bool
  out "Log Data Output (C)":bool
  out "Analog Channel-List":string
  out "Use Agilent?":bool
  out "Condition A":T2
  out "Update Heating Message":bool
  out "Test CompleteA":bool
  out "Test CompleteB":bool
  out "Test CompleteC":bool
  out "Test CompleteD":bool
  out "DAQ State":string
  out "Main State":string
  out "UI State":string
  in  "Scan Rate (Default)":T11=3.0 format="%.2f"
  out "K-Factor (Flow)":dbl
  out "Intellifaucet Type":string
  out "Disable Purge Pressurization A":bool
  out "DAQ Complete":bool
  out "Init Complete":bool
  out "DAQ":string[](array[string])
  out "Main Control":string[](array[string])
  in  "Debug":bool
  out "Module 4 Relay Status":T28
  out "Inficon Data":T53
  out "Manual HHV":bool
  in  "DAQ Timeout":i32=100
  out "Data Acquisition Steps Loop Count":i32
  out "MainLoop":i32
  out "DAQ Loop Rate":dbl format="%0.2f"
  out "Ritter Gas Drum Meter":bool
  in  "Meter Type":enum16{"Dry Meter", "Wet Meter"}(ring)
  in  "RLT Station Channels":T54
